vi "enumerateStaticDependencies.vi"(8 "error in (no error)":errorcluster, 11 "Measurement.PhotocurrentMapping":refnum<class "Measurement.PhotocurrentMapping.lvclass">) -> (0 "error out":errorcluster, 2 "Static Dependencies":refnum<class "Dependency.lvclass">[](array[class]), 3 "Measurement.PhotocurrentMapping out":refnum<class "Measurement.PhotocurrentMapping.lvclass">)   [LabVIEW 2017, in "Measurement.PhotocurrentMapping.lvclass"]
doc: "JKI State Machine Objects (SMO) 1.3.0.56\nJKI - JKI\nCopyright (c) 2017, JKI"
uses:
  Measurement.PhotocurrentMapping.lvclass
  <vilib>/JKI/JKI SMO/Dependency/Dependency.lvclass
  SMU/SMU.lvclass
  D:/Program Files (x86)/National Instruments/LabVIEW 2017/vi.lib/JKI/JKI SMO/SMO/SMO.lvclass
  LIA/LIA.lvclass
  Typedefs/Dependencies--Cluster.ctl
  XYStage/XYStage.lvclass
  Device/Device.lvclass
  Measurement/Measurement.lvclass
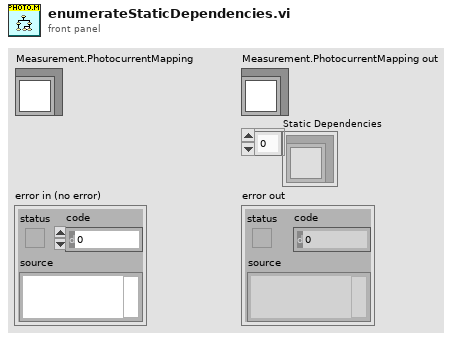
[diagram p1: front panel]
types:
  T1 = typedef "Measurement.PhotocurrentMapping.lvclass/Dependencies--Cluster.ctl" = cluster{"SMU":refnum<class "SMU.lvclass">, "LIA":refnum<class "LIA.lvclass">, "XYStage":refnum<class "XYStage.lvclass">}
  T2 = typedef "Measurement.PhotocurrentMapping.lvclass/Configuration--Cluster.ctl" = cluster{"Measurement.Type":T3, "Hardware":T4, "Measurement":T11}
  T3 = typedef "Measurement.lvclass/Measurement.Type--Enum.ctl" = enum16{"Free", "I/V Curve", "Wavelength sweeping", "Photocurrent mapping"}
  T4 = typedef "Measurement.PhotocurrentMapping.lvclass/Configuration.Hardware--Cluster.ctl" = cluster{"SMU":T5, "LIA":T7, "XYStage":T9}
  T5 = typedef "Measurement.lvclass/Configuration.SMU--Cluster.ctl" = cluster{"Enable":bool, "SMU Model":string, "Configuration":T6}
  T6 = typedef "SMU.lvclass/Configuration--Cluster.ctl" = cluster{"VISA Resource":string, "Channel":string}
  T7 = typedef "Measurement.lvclass/Configuration.LIA--Cluster.ctl" = cluster{"Enable":bool, "LIA Model":string, "Configuration":T8}
  T8 = typedef "LIA.lvclass/Configuration--Cluster.ctl" = cluster{"VISA Resource":string}
  T9 = typedef "Measurement.lvclass/Configuration.XYStage--Cluster.ctl" = cluster{"Enable":bool, "XYStage Model":string, "Configuration":T10}
  T10 = typedef "XYStage.lvclass/Configuration--Cluster.ctl" = cluster{"Serial Number":string, "X Axis":string, "Y Axis":string, "Real-World Units":string, "Counts per Unit":u32}
  T11 = typedef "Measurement.PhotocurrentMapping.lvclass/Configuration.Measurement--Cluster.ctl" = cluster{"X":T12, "Y":T12, "Accumulation":u16}
  T12 = typedef "Measurement.PhotocurrentMapping.lvclass/Configuration.Axis--Cluster.ctl" = cluster{"Start, units":dbl, "Stop, units":dbl, "Step, units":dbl}
  T13 = cluster{"SMU":refnum<class "SMU.lvclass">, "LIA":refnum<class "LIA.lvclass">, "XYStage":refnum<class "XYStage.lvclass">}
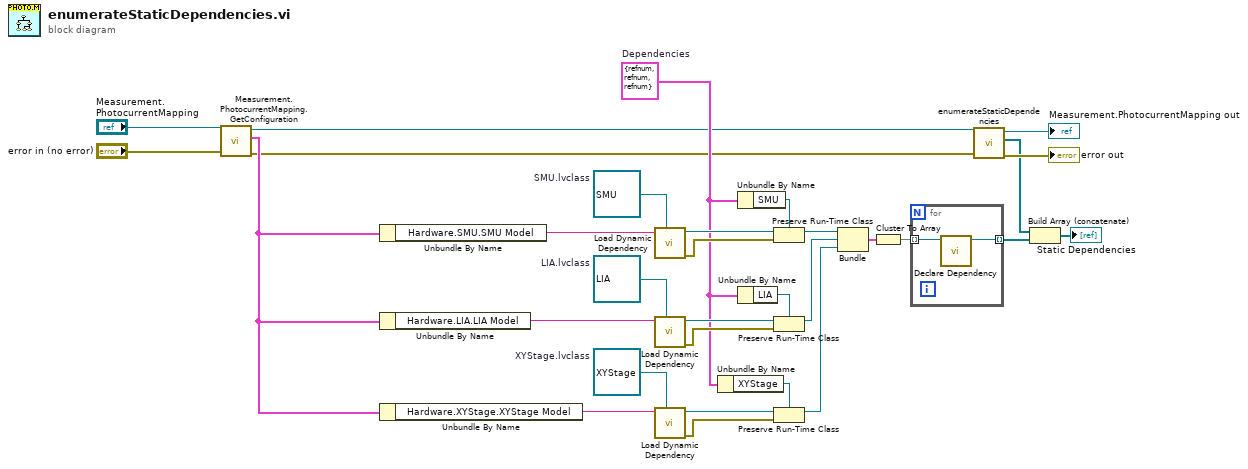
[diagram p0: block diagram]
diagram:
  w1 = refnum<class "XYStage.lvclass"> refnum  # XYStage.lvclass
  w7 = T1 {"SMU"=refnum, "LIA"=refnum, "XYStage"=refnum}  # Dependencies
  w21 = refnum<class "LIA.lvclass"> refnum  # LIA.lvclass
  w28 = refnum<class "SMU.lvclass"> refnum  # SMU.lvclass
  n1 = call "Measurement.PhotocurrentMapping.GetConfiguration.vi"("error in (no error)"="error in (no error)", "Measurement.PhotocurrentMapping"="Measurement.PhotocurrentMapping") -> ("error out"=w5:errorcluster, "Configuration"=w8:T2, "Measurement.PhotocurrentMapping out"=w6:refnum<class "Measurement.PhotocurrentMapping.lvclass">)  [unwired: 7 in]
  n2 = Unbundle By Name(w8) -> ("Hardware.SMU.SMU Model"=w29:string)
  n3 = Unbundle By Name(w8) -> ("Hardware.LIA.LIA Model"=w16:string)
  n4 = Unbundle By Name(w8) -> ("Hardware.XYStage.XYStage Model"=w15:string)
  n5 = call "Load Dynamic Dependency.vi"("SMO in"=w28, "Class Name"=w29) -> ("error out"=w25:errorcluster, "SMO out"=w26:refnum<class "SMU.lvclass">)  [unwired: 8 in]
  n6 = call "Load Dynamic Dependency.vi"("SMO in"=w21, "Class Name"=w16) -> ("error out"=w18:errorcluster, "SMO out"=w19:refnum<class "LIA.lvclass">)  [unwired: 8 in]
  n7 = call "Load Dynamic Dependency.vi"("SMO in"=w1, "Class Name"=w15) -> ("error out"=w13:errorcluster, "SMO out"=w14:refnum<class "XYStage.lvclass">)  [unwired: 8 in]
  n8 = Unbundle By Name(w7) -> ("XYStage"=w12:refnum<class "XYStage.lvclass">)
  n9 = Unbundle By Name(w7) -> ("SMU"=w27:refnum<class "SMU.lvclass">)
  n10 = Unbundle By Name(w7) -> ("LIA"=w20:refnum<class "LIA.lvclass">)
  n11 = Preserve Run-Time Class(object in=w26, error in=w25, 2:w27) -> (object out=w24:refnum<class "SMU.lvclass">)  [unwired: 1 out]
  n12 = Preserve Run-Time Class(object in=w19, error in=w18, 2:w20) -> (object out=w17:refnum<class "LIA.lvclass">)  [unwired: 1 out]
  n13 = Preserve Run-Time Class(object in=w14, error in=w13, 2:w12) -> (object out=w11:refnum<class "XYStage.lvclass">)  [unwired: 1 out]
  n14 = Bundle("SMU"=w24, "LIA"=w17, "XYStage"=w11) -> (w23:T13)  [unwired: 1 in]
  n15 = Cluster To Array(cluster=w23) -> (array=w22:refnum<class "Device.lvclass">[])
  n16 = for {
    tunnel: [w33] -> w4 mode=indexing
    tunnel: w22 -> [w32] mode=indexing
    n17 = call <vilib>:"Declare Dependency.vi"("Type"=w32) -> ("Dependency out"=w33:refnum<class "Dependency.lvclass">)  [unwired: 9 in, 1 out]
  }
  n18 = call-parent "enumerateStaticDependencies.vi"("error in (no error)"=w5, "SMO"=w6) -> ("error out"=→"error out":errorcluster, "Static Dependencies"=w3:refnum<class "Dependency.lvclass">[], "SMO out"=→"Measurement.PhotocurrentMapping out":refnum<class "Measurement.PhotocurrentMapping.lvclass">)  [unwired: 7 in]
  n19 = Build Array (concatenate)(w3, w4) -> (→"Static Dependencies":refnum<class "Dependency.lvclass">[])
